vi "E16_GraficoIntensidadCopia.vi"() -> ()   [LabVIEW 2026]
panel:
  out "Intensity Graph":dbl[][](graph)
  out "Array":dbl[][](array[numeric])
  in  "Columnas":i32
  in  "Filas":i32
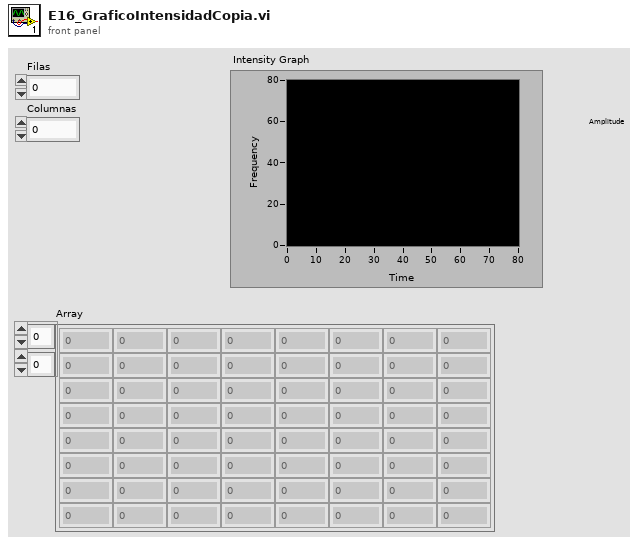
[diagram p1: front panel]
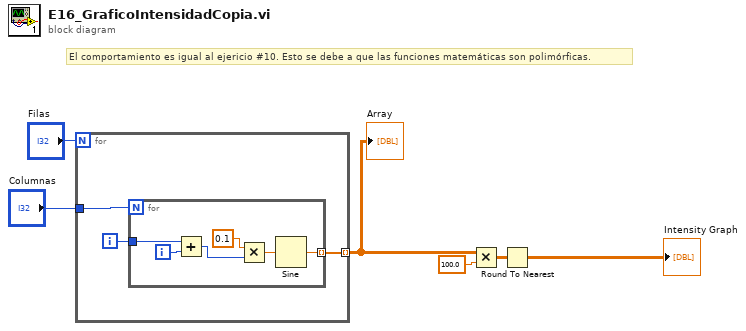
[diagram p0: block diagram]
diagram:
  # "El comportamiento es igual al ejericio #10. Esto se debe a que las funciones matemáticas son polimórficas."
  n1 = for {
    N: "Filas" -> [_]
    tunnel: "Columnas" -> [w9]
    tunnel: [w7] -> w3 mode=indexing
    i -> [w8]
    n2 = for {
      N: w9 -> [_]
      tunnel: w8 -> [w14]
      tunnel: [w10] -> w7 mode=indexing
      i -> [w15]
      n3 = Add(x=w14, y=w15) -> (x+y=w13:i32)
      n4 = Multiply(x=0.1, y=w13) -> (x*y=w11:dbl)
      n5 = Sine(x=w11) -> (sin(x)=w10:dbl)
    }
  }
  "Array" <- w3
  n6 = Multiply(x=w3, y=100.0) -> (x*y=w1:dbl[][])
  n7 = Round To Nearest(number=w1) -> (nearest integer value=→"Intensity Graph":dbl[][])
